vi "InternalErrorCodes.vi"() -> ()   [LabVIEW 2021, in "myRIOMetaDataObj.lvclass"]
uses:
  myRIOMetaDataObj.lvclass
panel:
  in  "Invalid IP or Hostname":string="The IP address or hostname is invalid."
  in  "Timeout":string="The operation timed out."
  in  "ShutdownTarget":string="Cannot connect to the %s because the %s is turned off or the IP address is incorrect."
  in  "EmptyIP":string="The IP address or hostname is empty."
  in  "SearchingTarget":string="Searching for targets ..."
  in  "ConnectTargetByIP":string="Connecting to the target ..."
  in  "Full Zero IP Address":string="The IP address cannot be 0.0.0.0."
  in  "Not Supported Target":string="The target you specified is not %s %s device. "
  in  "No Target":string="No %s devices found."
  in  "Select Target":string="Please select %s %s device. "
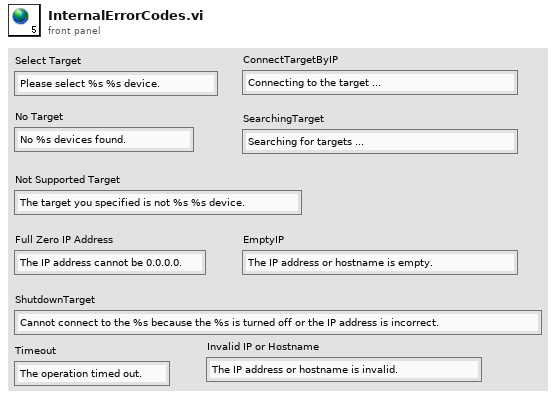
[diagram p1: front panel]
diagram:
